vi "OpenInterface.vi"(8 "error in (no error)":errorcluster) -> (0 "error out":errorcluster, 1 "specific error cleared?":bool, 2 "handle":i32)   [LabVIEW 2014]
uses:
  Program Files (x86)/CAEN/Comm/labview/CAENComm.lvlib
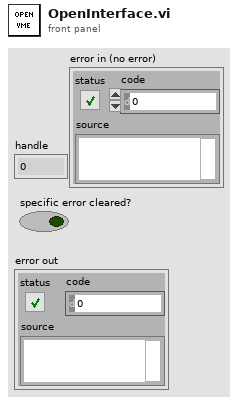
[diagram p1: front panel]
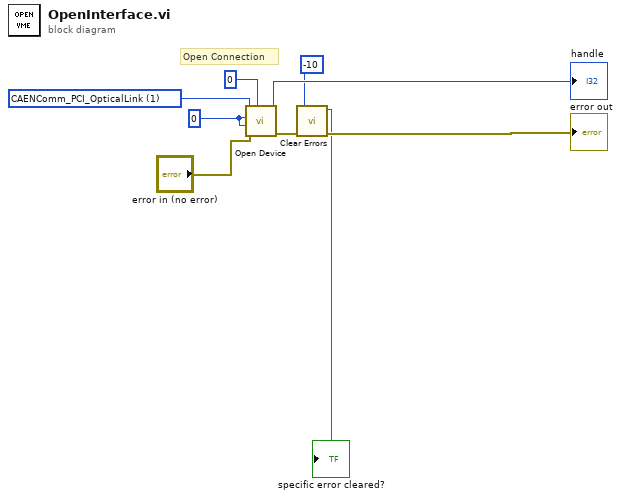
[diagram p0: block diagram]
diagram:
  w2 = 0 ("LinkNum")
  w1 = u32 1 items=["CAENComm_USB", "CAENComm_PCI_OpticalLink", "CAENComm_PCIE_OpticalLink", "CAENComm_PCIE"] ("LinkType")
  # "Open Connection"
  n1 = call "Open Device.vi"("VMEBaseAddress"=u32 0, "error in (no error)"="error in (no error)", "ConetNode"=w2, "LinkNum"=w2, "LinkType"=w1) -> ("error out"=w5:errorcluster, "handle"=→"handle":i32)  [unwired: 5 in]
  n2 = call <vilib>:"Clear Errors.vi"("error in (no error)"=w5, "specific error code to clear (0: all)"=-10) -> ("error out"=→"error out":errorcluster, "specific error cleared?"=→"specific error cleared?":bool)  [unwired: 4 in]
